vi "Write Holding Registers_Cached.vi"(8 "error in (no error)":errorcluster, 9 "Modbus Data Block":u16[](array[numeric]), 10 "Modbus Address":u16, 11 "MB PLC in":refnum<class "MB PLC Client.lvclass">) -> (0 "error out":errorcluster, 3 "MB PLC out":refnum<class "MB PLC Client.lvclass">)   [LabVIEW 2018, in "MB PLC Client.lvlib" / "MB PLC Client.lvclass"]
uses:
  MB PLC Client.lvclass
  MB PLC Client.lvclass/MB PLC Client.ctl
  Data/MB Data Block.lvclass
  <vilib>/Plasmionique/MB Master/MB Master.lvlib
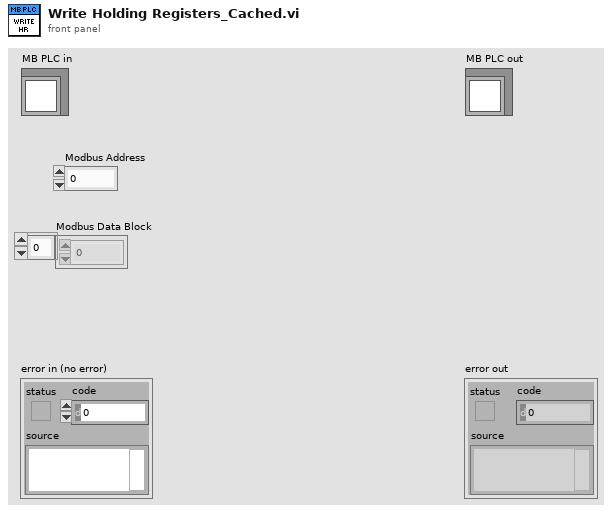
[diagram p1: front panel]
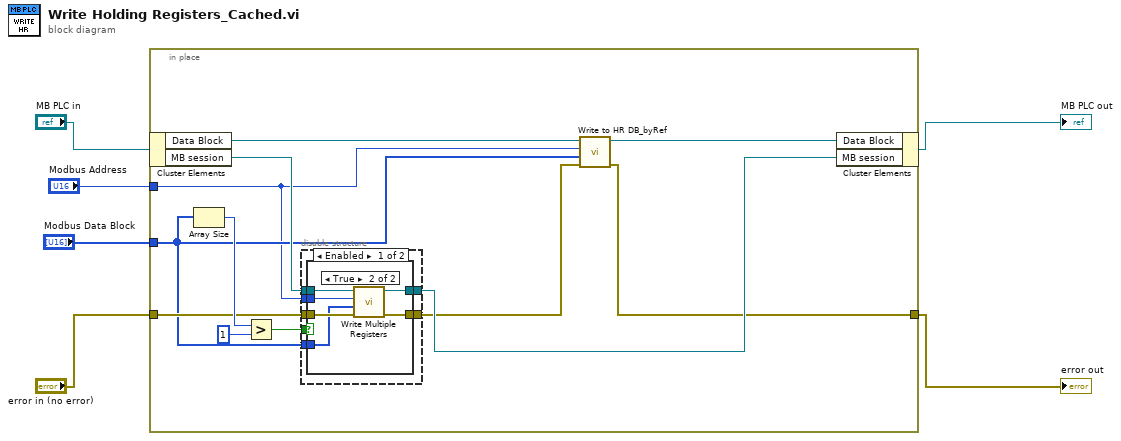
[diagram p0: block diagram]
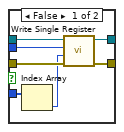
[diagram p2: hidden frame]
diagram:
  n1 = in-place {
    in-place-border: "Modbus Address" -> [w9]
    in-place-border: "Modbus Data Block" -> [w10]
    in-place-border: "error in (no error)" -> [w16]
    in-place-border: [w7] -> w1
    n2 = in-place-cluster #1("MB PLC in") -> ("Data Block"=w12:refnum<data-value>, "MB session"=w15:refnum<class "MB_Master.lvclass">)
    n3 = Array Size(array=w10) -> (size(s)=w18:i32)
    n4 = Greater?(x=w18, y=1) -> (0:w13:bool)
    n5 = disable-structure shown="Enabled" {
      disable-tunnel: [w25 w39] -> w8
      disable-tunnel: w16 -> [w24 w39]
      disable-tunnel: w15 -> [w23 w40]
      disable-tunnel: [w22 w40] -> w14
      disable-tunnel: w9 -> [w21 _]
      disable-tunnel: w10 -> [w20 _]
      disable-tunnel: w13 -> [w19 _]
      frame Enabled {
        n6 = case shown="True" w19 {
          tunnel: [w32 w35] -> w25
          tunnel: w24 -> [w31 w36]
          tunnel: w23 -> [w30 w38]
          tunnel: [w29 w37] -> w22
          tunnel: w21 -> [w28 w34]
          tunnel: w20 -> [w27 w33]
          frame False {
            n7 = Index Array(array=w27) -> (element=w26:u16)  [unwired: 1 in]
            n8 = call <vilib>:"Write Single Register.vi"("error in (no error)"=w31, "value"=w26, "address"=w28, "MB session in"=w30) -> ("error out"=w32:errorcluster, "MB session out"=w29:refnum<class "MB_Master.lvclass">)  [unwired: 6 in]
          }
          frame True {
            n9 = call <vilib>:"Write Multiple Registers.vi"("error in (no error)"=w36, "values"=w33, "starting address"=w34, "MB session in"=w38) -> ("error out"=w35:errorcluster, "MB session out"=w37:refnum<class "MB_Master.lvclass">)  [unwired: 6 in]
          }
        }
      }
      frame Disabled {
      }
    }
    n10 = call "Write to HR DB_byRef.vi"("error in (no error)"=w8, "Values"=w10, "Modbus Address"=w9, "Cache Ref in"=w12) -> ("error out"=w7:errorcluster, "Cache Ref out"=w11:refnum<data-value>)  [unwired: 6 in]
    n11 = in-place-cluster #1("Data Block"=w11, "MB session"=w14) -> (→"MB PLC out":refnum<class "MB PLC Client.lvclass">)
  }
  "error out" <- w1
